vi "Get Logger Status.vi"(8 "error in (no error)":errorcluster, 11 "LoggerReference in":refnum<class "LoggerReference.lvclass">) -> (0 "error out":errorcluster, 1 "Logger Running?":bool, 2 "Logger Instantiated?":bool, 3 "LoggerReference out":refnum<class "LoggerReference.lvclass">)   [LabVIEW 2020, in "Composed Log.lvlib" / "LoggerReference.lvclass"]
uses:
  <vilib>/gpm_packages/@cs/event-logger/Source/Composed Log/LoggerReference/LoggerReference.lvclass
  <vilib>/gpm_packages/@cs/event-logger/Source/Composed Log/LoggerReference/LoggerReference.lvclass/LoggerReference.ctl
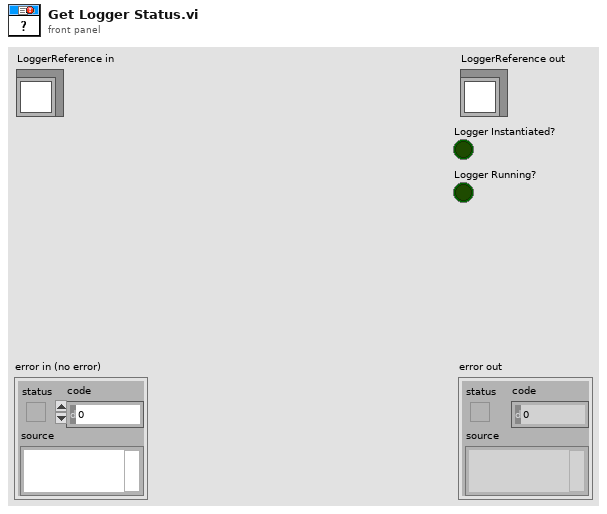
[diagram p1: front panel]
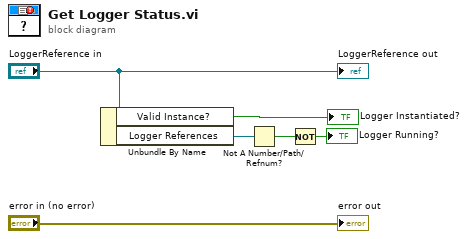
[diagram p0: block diagram]
diagram:
  n1 = Unbundle By Name("LoggerReference in") -> ("Valid Instance?"=→"Logger Instantiated?":bool, "Logger References"=w3:refnum<data-value>)
  n2 = Not A Number/Path/Refnum?(number/path/refnum=w3) -> (NaN/Path/Refnum?=w2:bool)
  n3 = Not(x=w2) -> (.not. x?=→"Logger Running?":bool)
  "error out" <- "error in (no error)"
  "LoggerReference out" <- "LoggerReference in"
